vi "TUNA init IR sensor.vi"() -> (0 "IR Sensors":T1(array[cluster]))   [LabVIEW 2014]
doc: "This vi initiates the IR sensors as an array of clusters with Name, local angle direction, and distance reading. A reading of 0.0 is meant to be no object found."
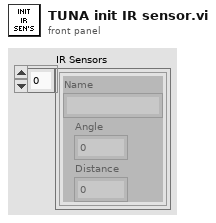
[diagram p1: front panel]
types:
  T1 = cluster{"Name":string, "Angle":dbl, "Distance":dbl}[]
  T2 = cluster{"Name":string, "Angle":dbl, "Distance":dbl}
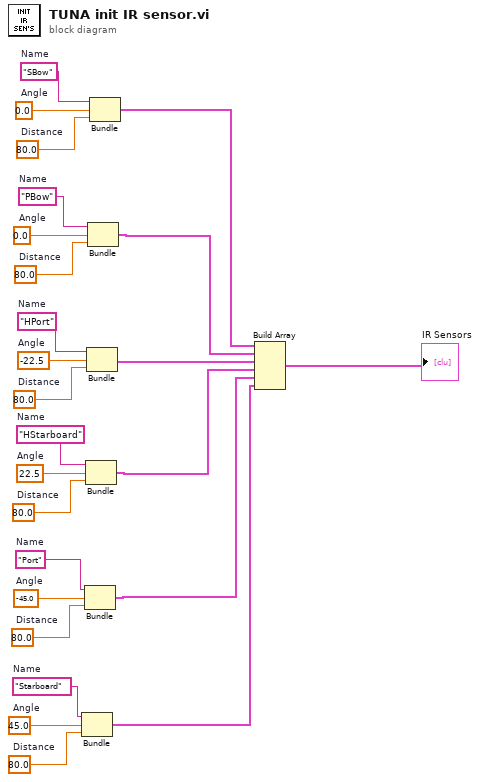
[diagram p0: block diagram]
diagram:
  w2 = 80.0  # Distance
  w4 = 45.0  # Angle
  w3 = "Starboard"  # Name
  w11 = 80.0  # Distance
  w13 = -45.0  # Angle
  w12 = "Port"  # Name
  w14 = 80.0  # Distance
  w16 = 22.5  # Angle
  w15 = "HStarboard"  # Name
  w17 = 80.0  # Distance
  w19 = -22.5  # Angle
  w18 = "HPort"  # Name
  w20 = 80.0  # Distance
  w22 = 0.0  # Angle
  w21 = "PBow"  # Name
  w23 = 80.0  # Distance
  w25 = 0.0  # Angle
  w24 = "SBow"  # Name
  n1 = Bundle("Name"=w3, "Angle"=w4, "Distance"=w2) -> (w1:T2)  [unwired: 1 in]
  n2 = Bundle("Name"=w12, "Angle"=w13, "Distance"=w11) -> (w6:T2)  [unwired: 1 in]
  n3 = Bundle("Name"=w15, "Angle"=w16, "Distance"=w14) -> (w7:T2)  [unwired: 1 in]
  n4 = Bundle("Name"=w18, "Angle"=w19, "Distance"=w17) -> (w8:T2)  [unwired: 1 in]
  n5 = Bundle("Name"=w21, "Angle"=w22, "Distance"=w20) -> (w9:T2)  [unwired: 1 in]
  n6 = Bundle("Name"=w24, "Angle"=w25, "Distance"=w23) -> (w10:T2)  [unwired: 1 in]
  n7 = Build Array(w10, w9, w8, w7, w6, w1) -> (→"IR Sensors":T1)
